vi "Get All Drives Info(冲突时的文件备份2013-03-27 14-09-21).vi"(8 "error in (no error)":errorcluster caption="错误输入（无错误）") -> (0 "error out":errorcluster caption="错误输出", 3 "Drives":T1[](array[typedef]) {"DriveType" items=["Unknown", "NoRootDirectory", "Removable", "Fixed", "Network", "CDRom", "Ram"]})   [LabVIEW 2012, in "DriveInfo.lvclass"]
uses:
  DriveInfo.lvclass
  Info.ctl
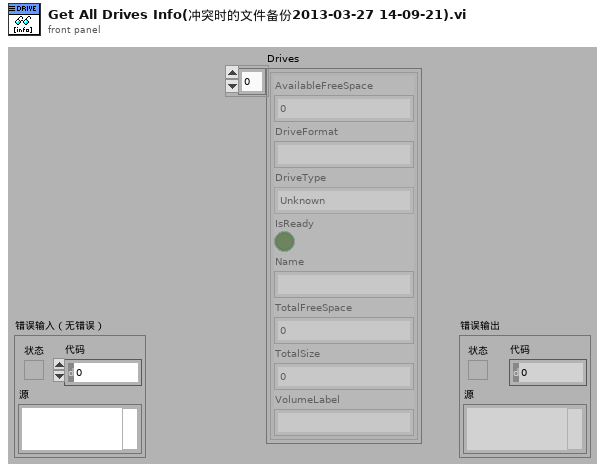
[diagram p1: front panel]
types:
  T1 = typedef "DriveInfo.lvclass/Info.ctl" = cluster{"AvailableFreeSpace":i64, "DriveFormat":string, "DriveType":i32, "IsReady":bool, "Name":string, "TotalFreeSpace":i64, "TotalSize":i64, "VolumeLabel":string}
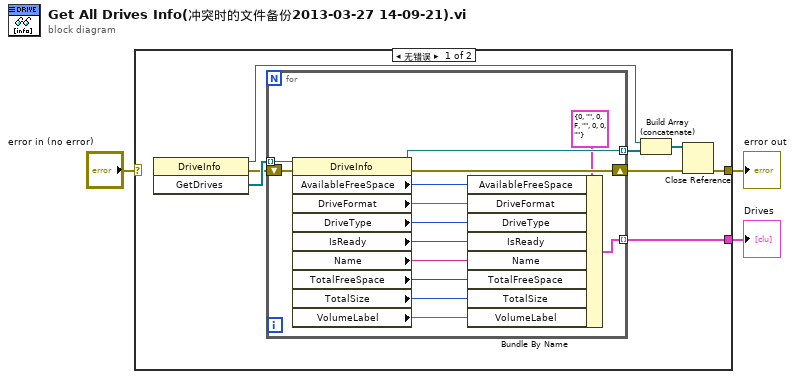
[diagram p0: block diagram]
diagram:
  n1 = case shown="无错误" "error in (no error)" {
    selector: "error in (no error)" -> [_ w26]
    tunnel: [w9 _] -> w2
    tunnel: [w5 w26] -> w1
    frame No Error {
      n2 = invoke class="DriveInfo" method="GetDrives"() -> (reference out=w7:refnum<k24>, error out=w10:errorcluster, "GetDrives"=w11:refnum<k24>[])  [unwired: 3 in]
      n3 = for {
        tunnel: w11 -> [w25] mode=indexing
        shift-right: [w23] -> w6
        shift-left: w10 -> [w24]
        tunnel: [w22] -> w8 mode=indexing
        tunnel: [w20] -> w9 mode=indexing
        n4 = property class="DriveInfo"(reference=w25, error in=w24) -> (reference out=w22:refnum<k24>, error out=w23:errorcluster, "AvailableFreeSpace"=w19:i64, "DriveFormat"=w18:string, "DriveType"=w17:i32, "IsReady"=w16:bool, "Name"=w15:string, "TotalFreeSpace"=w14:i64, "TotalSize"=w13:i64, "VolumeLabel"=w12:string)
        n5 = Bundle By Name(cluster=T1 {"AvailableFreeSpace"=0, "DriveFormat"="", "DriveType"=0, "IsReady"=FALSE, "Name"="", "TotalFreeSpace"=0, "TotalSize"=0, "VolumeLabel"=""} ("DriveInfo"), "AvailableFreeSpace"=w19, "DriveFormat"=w18, "DriveType"=w17, "IsReady"=w16, "Name"=w15, "TotalFreeSpace"=w14, "TotalSize"=w13, "VolumeLabel"=w12) -> (w20:T1)
      }
      n6 = Build Array (concatenate)(w7, w8) -> (w4:refnum<k24>[])
      n7 = Close Reference(reference=w4, error in (no error)=w6) -> (error out=w5:errorcluster)
    }
    frame Error {
    }
  }
  "error out" <- w1
  "Drives" <- w2
